vi "单元格位置.vi"(8 "错误输入（无错误）":errorcluster, 10 "单元格位置":T1, 11 "Table输入":refnum<vi>) -> (0 "错误输出":errorcluster, 2 "单元格大小":T2, 3 "Table输出":refnum<vi>)   [LabVIEW 2014, in "表格.lvlib"]
uses:
  <vilib>/Utility/miscctls.llb/LVRowAndColumnTypeDef.ctl
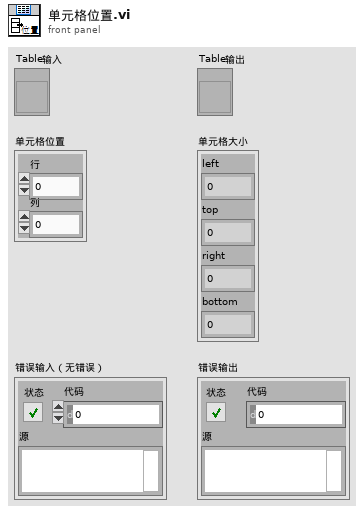
[diagram p1: front panel]
types:
  T1 = typedef "LVRowAndColumnTypeDef.ctl" = cluster{"Row":i32, "Column":i32}
  T2 = cluster{"left":i16, "top":i16, "right":i16, "bottom":i16}
  T3 = typedef "LVPositionTypeDef.ctl" = cluster{"Left":i32, "Top":i32}
  T4 = typedef "LVBoundsTypeDef.ctl" = cluster{"Width":u32, "Height":u32}
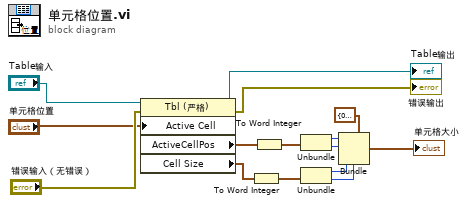
[diagram p0: block diagram]
diagram:
  n1 = property on="Property Node" class="Tbl (严格)"(reference="Table输入", error in="错误输入（无错误）", "Active Cell"="单元格位置") -> (reference out=→"Table输出":refnum<vi>, error out=→"错误输出":errorcluster, "ActiveCellPos"=w6:T3, "Cell Size"=w7:T4)
  n2 = To Word Integer(number=w7) -> (16bit integer=w9:cluster{"Width":i16, "Height":i16})
  n3 = To Word Integer(number=w6) -> (16bit integer=w1:cluster{"Left":i16, "Top":i16})
  n4 = Unbundle(w1) -> ("Left"=w5:i16, "Top"=w4:i16)
  n5 = Unbundle(w9) -> ("Width"=w3:i16, "Height"=w2:i16)
  n6 = Bundle(cluster=T2 {"left"=0, "top"=0, "right"=0, "bottom"=0} ("Cell Rect Out"), "left"=w5, "top"=w4, "right"=w3, "bottom"=w2) -> (→"单元格大小":T2)
